vi "SetStopSwitchLimits.vi"(0 "handle in":i32, 1 "UnitAddress(0)":u16, 2 "Channel(0)":u8, 5 "error in":errorcluster, 7 "Stopswitch Limits":T1={"MinLeft(0)"=0, "MaxRight(1023)"=1023}) -> (14 "handle out":i32, 19 "error out":errorcluster)   [LabVIEW 2014, in "Sixpack - Driver.lvlib"]
doc: "Uber ein Potentiometer oder eine Widerstandsbeschaltung von zwei Endschaltern, kann uber den Analogeingang jedes Motors ein Stopp (hart oder weich) ausgelost werden. Die Spannung am Analogeingang soll in Fahrtrichtung rechts ansteigen. Der gemessene Wert wird in Abhangigkeit von der Fahrtrichtung uberpruft. Wenn eine Stopp-Bedingung eintritt, wird der Motor sofort angehalten. \n\nDie Werte fur MinLeft bzw. MaxRight errechnen sich uber die Formel Wert = (Max.|Min.)-Spannung * (5V / 1023).\n\nIst das Flag MT_STOPSOFT gesetzt, so wird mit der durch AMax eingestellten Beschleunigung abgebremst. \n\n(Achtung: Falls vor dem Stillstand die Stopp.Bedingung nicht mehr gilt, wird weitergefahren)\nWenn MT_STOPSOFT nicht gesetzt ist halt der Motor abrupt an, so dass die genaue Motorposition fur weitere Fahrten verloren gehen kann. Deshalb wird zusatzlich eine Referenzfahrt gestartet, es sei denn, das Flag MT_STOPNOREF ist gesetzt. Ist das Flag MT_STOPNULL gesetzt, fungiert der Nullschalter selbst gleichzeitig auch als Endabschalter an seiner Seite.\n\nCMD $31\nChannel: (0...7)\nMinLeft: Analogwert Minimum fur Stopp links (0=keine Funktion, d.h. linker Endschalter deaktiviert)\nMaxRight: Analogwert Maximum fur Stopp rechts (>1023=keine Funktion, d.h. rechter Endschalter deaktiviert)"
uses:
  Sixpack - Driver.lvlib
  Stopswitch Limits.ctl
  DLL/PackDLL.dll
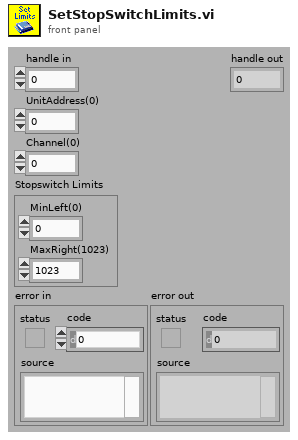
[diagram p1: front panel]
types:
  T1 = typedef "Sixpack - Driver.lvlib/Stopswitch Limits.ctl" = cluster{"MinLeft(0)":u16, "MaxRight(1023)":u16}
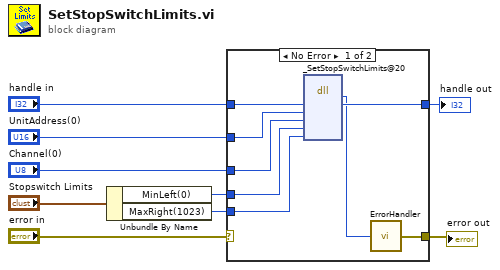
[diagram p0: block diagram]
diagram:
  n1 = Unbundle By Name("Stopswitch Limits") -> ("MinLeft(0)"=w2:u16, "MaxRight(1023)"=w1:u16)
  n2 = case shown="No Error" "error in" {
    selector: "error in" -> [_ w18]
    tunnel: "handle in" -> [w17 w19]
    tunnel: [w16 w19] -> w8
    tunnel: "UnitAddress(0)" -> [w15 _]
    tunnel: "Channel(0)" -> [w14 _]
    tunnel: w2 -> [w13 _]
    tunnel: w1 -> [w12 _]
    tunnel: [w10 w18] -> w5
    frame No Error {
      n3 = dll-call lib="D:/CS-Source/LV2014/GPL/instr.lib/SixPack/PackDLL/DLL/PackDLL.dll" fn="_SetStopSwitchLimits@20" label="SetStopSwitchLimits"("HANDLE"=w17, "UnitAddress"=w15, "Channel"=w14, "MinLeft"=w13, "MaxRight"=w12) -> ("BOOLEAN"=w11:i8, "HANDLE"=w16:i32)  [unwired: 7 in, 2 out]
      n4 = call "ErrorHandler.vi"("BOOLEAN"=w11) -> ("error out"=w10:errorcluster)
    }
    frame Error {
    }
  }
  "handle out" <- w8
  "error out" <- w5
